vi "Interpolate 1D Array Main Page.vi"(8 "error in (no error)":errorcluster, 11 "Node Ptr":T5 format="%.0x") -> (0 "error out":errorcluster)   [LabVIEW 2011, in "Interpolate 1D Array Custom Device.lvlib"]
uses:
  Interpolate 1D Array Custom Device.lvlib
  <vilib>/NI Veristand/Custom Device API/Custom Device Item Ref.ctl
  Interpolate Options.ctl
  File Dependency Control.ctl
  <vilib>/NI Veristand/Custom Device API/Path Type.ctl
  Delimiter Control.ctl
  Spreadsheet Info.ctl
  <vilib>/NI Veristand/Custom Device API/Custom Device File Dependency.ctl
  <vilib>/NI Veristand/Custom Device API/Path Specification.ctl
  <vilib>/NI Veristand/Custom Device API/Custom Device Supported Target.ctl
  Global Property Names.vi
  <vilib>/NI Veristand/Custom Device API/Get Item Property (Variant).vi
  <vilib>/NI Veristand/Custom Device API/Set Item Property (Variant).vi
  <vilib>/NI Veristand/Custom Device API/Set Item Property (Path).vi
  <vilib>/NI Veristand/Custom Device API/Custom Device API.lvlib
panel:
  in  "Delimiter":T1
  in  "Dependency":T2={"Source"={"Local Path"=path "", "Type"=enum."Absolute"}, "RT Path"=path "", "Force Download File?"=TRUE}
  in  "Interpolate Options":T4={"method"=1, "ntimes"=1, "X is monotonic"=FALSE} {"method" items=["nearest", "linear", "spline", "cubic Hermite", "Lagrange"]}
  in  "Row Offset":dbl
  in  "Header":cluster{"Section Name":string}={"Section Name"="Custom Device Item Settings"}
  in  "Description":string
  in  "Name":string
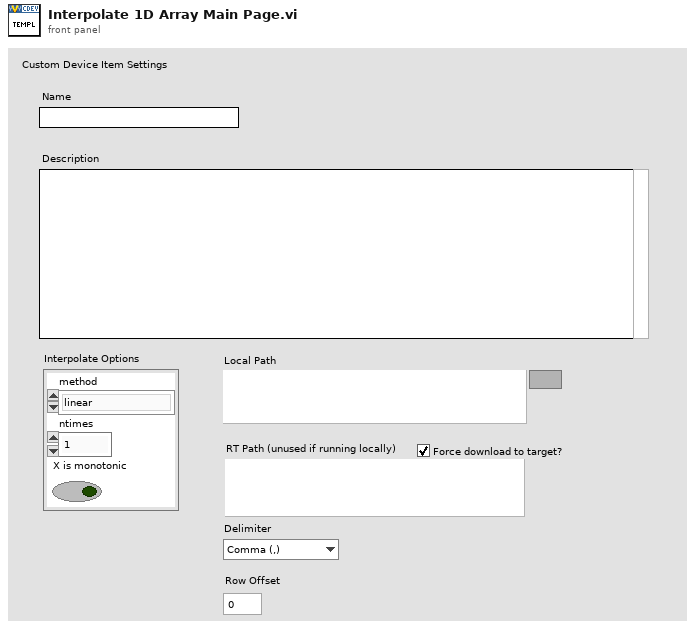
[diagram p1: front panel]
types:
  T1 = typedef "Interpolate 1D Array Custom Device.lvlib/Delimiter Control.ctl" = enum16{"Comma (,)", "Tab (\\t)"}
  T2 = typedef "Interpolate 1D Array Custom Device.lvlib/File Dependency Control.ctl" = cluster{"Source":cluster{"Local Path":path, "Type":T3}, "RT Path":path, "Force Download File?":bool}
  T3 = typedef "Custom Device API.lvlib/Path Type.ctl" = enum16{"Absolute", "To Base", "To Common Data Dir", "To Application Data Dir"}
  T4 = typedef "Interpolate 1D Array Custom Device.lvlib/Interpolate Options.ctl" = cluster{"method":i32, "ntimes":i32, "X is monotonic":bool}
  T5 = typedef "Custom Device API.lvlib/Custom Device Item Ref.ctl" = u64
  T6 = typedef "Interpolate 1D Array Custom Device.lvlib/Spreadsheet Info.ctl" = cluster{"Delimiter":string, "Row Offset":dbl}
  T7 = typedef "Custom Device API.lvlib/Custom Device File Dependency.ctl" = cluster{"Source":T8, "RT Destination":path, "ForceDownload?":bool, "SupportedTarget":T9, "Version":string}
  T8 = typedef "Custom Device API.lvlib/Path Specification.ctl" = cluster{"Path":path, "Type":T3}
  T9 = typedef "Custom Device API.lvlib/Custom Device Supported Target.ctl" = enum16{"All", "PharLap", "VxWorks", "Windows", "PharLap & Windows", "PharLap & VxWorks", "VxWorks & Windows"}
  T10 = typedef "Custom Device API.lvlib/Custom Device Item Info.ctl" = cluster{"Name":string, "Is Channel":bool, "GUID":string}
  T11 = typedef "Custom Device API.lvlib/Custom Device Commands.ctl" = enum16{"Default", "Item renamed", "Shutdown", "Dynamic button pressed"}
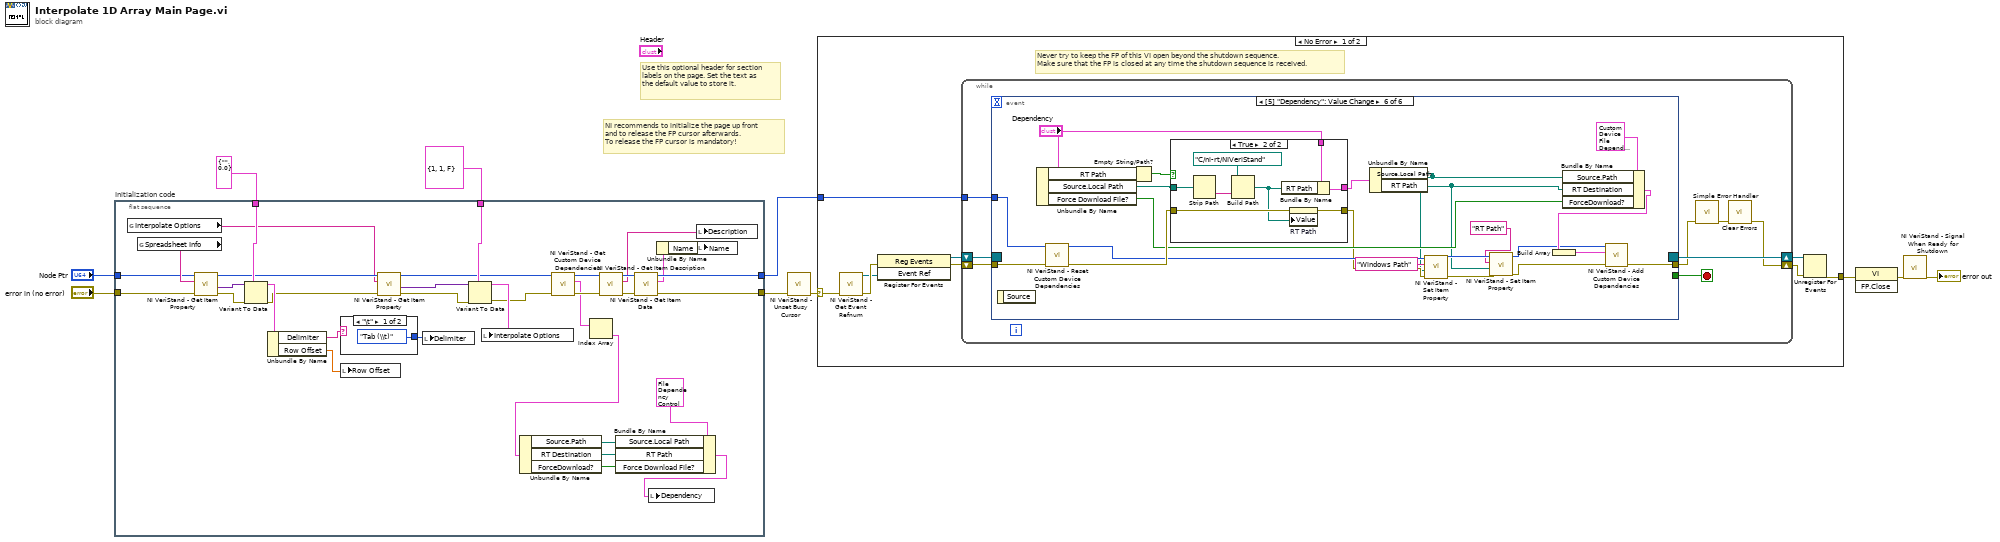
[diagram p0: block diagram]
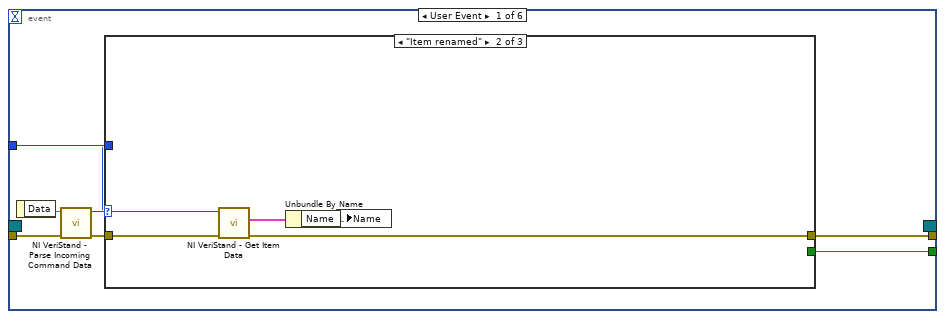
[diagram p2: hidden frame]
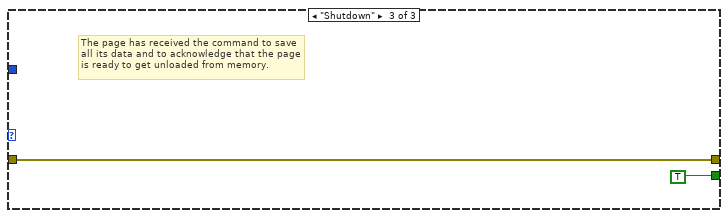
[diagram p4: hidden frame]
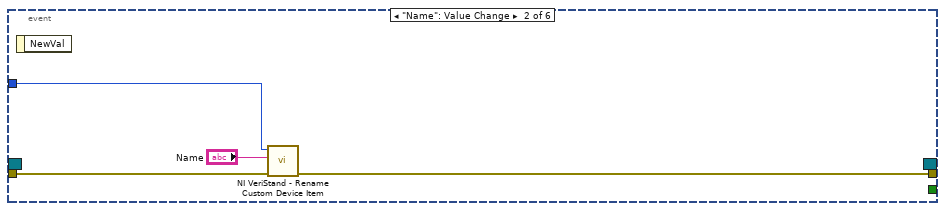
[diagram p5: hidden frame]
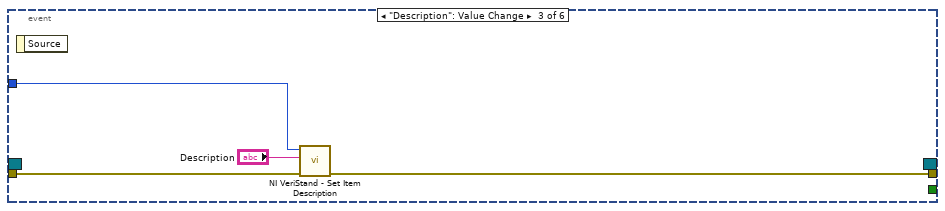
[diagram p6: hidden frame]
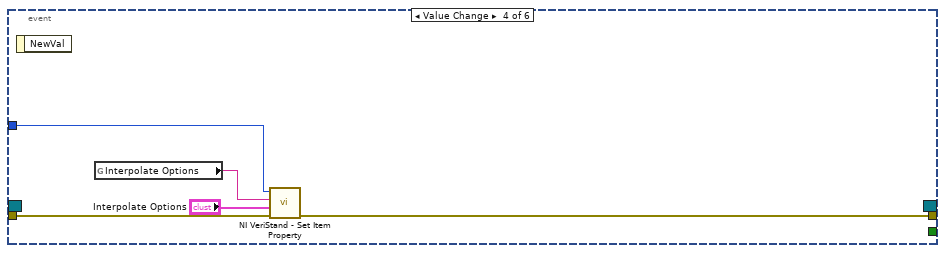
[diagram p7: hidden frame]
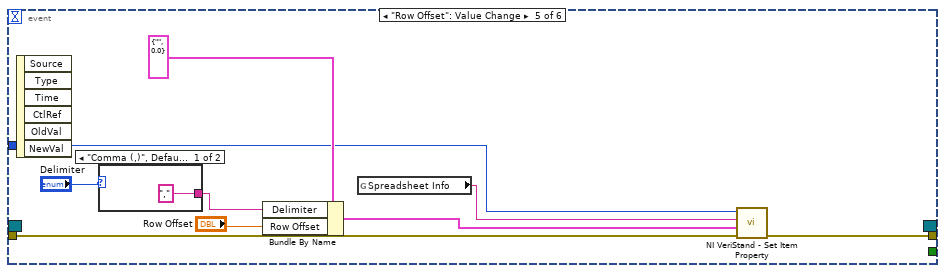
[diagram p8: hidden frame]
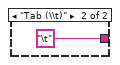
[diagram p9: hidden frame]
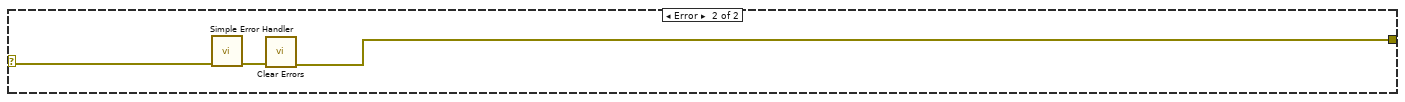
[diagram p11: hidden frame]
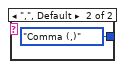
[diagram p12: hidden frame]
diagram:
  # "Use this optional header for section labels on the page. Set the text as the default value to store it."
  # "NI recommends to initialize the page up front\nand to release the FP cursor afterwards.\nTo release the FP cursor is mandatory!"
  n1 = flat-sequence "Initialization code" {
    tunnel: "error in (no error)" -> [w36]
    tunnel: "Node Ptr" -> [w37]
    tunnel: [w39] -> w8
    tunnel: [w45] -> w5
    tunnel: T6 {"Delimiter"="", "Row Offset"=0.0} ("Spreadsheet Info") -> [w33]
    tunnel: T4 {"method"=1, "ntimes"=1, "X is monotonic"=FALSE} ("Interpolate Options") -> [w26]
    frame #0 {
      n2 = global read "Global Property Names.vi" "Interpolate Options"() -> (w24:string)
      n3 = global read "Global Property Names.vi" "Spreadsheet Info"() -> (w38:string)
      n4 = call-poly <vilib>:"NI VeriStand - Get Item Property.vi"("error in (no error)"=w36, "Property Name"=w38, "Item Ref in"=w37) -> ("error out"=w34:errorcluster, "Value"=w35:variant, "Item Ref out"=w30:T5)  [unwired: 5 in, 1 out]
      n5 = Variant To Data(error in=w34, type=w33, Variant=w35) -> (data=w32:T6, error out=w29:errorcluster)
      n6 = Unbundle By Name(w32) -> ("Delimiter"=w18:string, "Row Offset"=w31:dbl)
      n7 = local write "Row Offset"(w31) -> ()
      n8 = case shown="\"\\t\"" w18 {
        tunnel: [Delimiter_Control."Tab (\\t)" ("Delimiter") Delimiter_Control."Comma (,)" ("Delimiter")] -> w17
        frame "\t" {
        }
        frame ",", Default {
        }
      }
      n9 = call-poly <vilib>:"NI VeriStand - Get Item Property.vi"("error in (no error)"=w29, "Property Name"=w24, "Item Ref in"=w30) -> ("error out"=w28:errorcluster, "Value"=w27:variant, "Item Ref out"=w22:T5)  [unwired: 5 in, 1 out]
      n10 = local write "Delimiter"(w17) -> ()
      n11 = Variant To Data(error in=w28, type=w26, Variant=w27) -> (data=w25:T4, error out=w23:errorcluster)
      n12 = local write "Interpolate Options"(w25) -> ()
      n13 = call <vilib>:"NI VeriStand - Get Custom Device Dependencies.vi"("error in (no error)"=w23, "Device Ref in"=w22) -> ("error out"=w20:errorcluster, "Dependencies"=w19:T7[], "Device Ref out"=w21:T5)  [unwired: 7 in]
      n14 = Index Array(array=w19) -> (element=w13:T7)  [unwired: 1 in]
      n15 = Unbundle By Name(w13) -> ("Source.Path"=w16:path, "RT Destination"=w14:path, "ForceDownload?"=w15:bool)
      n16 = call <vilib>:"NI VeriStand - Get Item Description.vi"("error in (no error)"=w20, "Item Ref in"=w21) -> ("error out"=w42:errorcluster, "Description"=w43:string, "Item Ref out"=w44:T5)  [unwired: 7 out]
      n17 = Bundle By Name(cluster=T2 {"Source"={"Local Path"=path "", "Type"=enum."Absolute"}, "RT Path"=path "", "Force Download File?"=TRUE} ("Dependency"), "Source.Local Path"=w16, "RT Path"=w14, "Force Download File?"=w15) -> (w12:T2)
      n18 = call <vilib>:"NI VeriStand - Get Item Data.vi"("error in (no error)"=w42, "Item Ref in"=w44) -> ("error out"=w39:errorcluster, "Item Info"=w41:T10, "Item Ref out"=w45:T5)  [unwired: 7 out]
      n19 = local write "Dependency"(w12) -> ()
      n20 = Unbundle By Name(w41) -> ("Name"=w40:string)
      n21 = local write "Description"(w43) -> ()
      n22 = local write "Name"(w40) -> ()
    }
  }
  n23 = call <vilib>:"NI VeriStand - Unset Busy Cursor.vi"("error in (no error)"=w8) -> ("error out"=w7:errorcluster)  [unwired: 10 out]
  n24 = case shown="No Error" w7 {
    selector: w7 -> [w48 w139]
    tunnel: [w53 w137] -> w10
    tunnel: w5 -> [w49 _]
    frame No Error {
      # "Never try to keep the FP of this VI open beyond the shutdown sequence.\nMake sure that the FP is closed at any time the shutdown sequence is received."
      n25 = call <vilib>:"NI VeriStand - Get Event Refnum.vi"("error in (no error)"=w48) -> ("error out"=w56:errorcluster, "Event Ref"=w52:refnum<user-event>)  [unwired: 9 out]
      n26 = register-events(error in=w56, w52) -> (reference out=w50:refnum<event-registration>, error out=w51:errorcluster)  [unwired: 1 in]
      n27 = while {
        tunnel: w49 -> [w60]
        shift-right: [w57] -> w54
        shift-left: w51 -> [w63]
        shift-right: [w64] -> w55
        shift-left: w50 -> [w62]
        stop <- w61 stop-if-true
        n28 = event shown="[5] \"Dependency\": Value Change" {
          selector: w62 -> [_ _ _ _ _ _]
          dyn-events: [_ _ _ _ _ _] -> w64
          timeout: _ -> [_ _ _ _ _ _]
          tunnel: w63 -> [w71 w83 w86 w91 w100 w123]
          tunnel: [w67 _ _ _ _ _] -> w61
          tunnel: [w66 w82 w85 w90 w99 w124] -> w59
          tunnel: w60 -> [w65 w81 w87 w92 w98 w126]
          event User Event {
            n29 = event-data() -> ("Data"=w70:string)  [unwired: 1 out]
            n30 = call <vilib>:"NI VeriStand - Parse Incoming Command Data.vi"("error in (no error)"=w71, "Incoming data"=w70) -> ("error out"=w69:errorcluster, "Action"=w68:T11)  [unwired: 8 out]
            n31 = case shown="\"Item renamed\"" w68 {
              tunnel: w69 -> [w72 w77 w78]
              tunnel: [_ _ TRUE] -> w67
              tunnel: [w72 w74 w78] -> w66
              tunnel: w65 -> [_ w76 _]
              frame "Default", Default {
              }
              frame "Item renamed" {
                n32 = call <vilib>:"NI VeriStand - Get Item Data.vi"("error in (no error)"=w77, "Item Ref in"=w76) -> ("error out"=w74:errorcluster, "Item Info"=w75:T10)  [unwired: 8 out]
                n33 = Unbundle By Name(w75) -> ("Name"=w73:string)
                n34 = local write "Name"(w73) -> ()
              }
              frame "Shutdown" {
                # "The page has received the command to save all its data and to acknowledge that the page is ready to get unloaded from memory."
              }
            }
          }
          event "Name": Value Change {
            n35 = event-data() -> ()  [unwired: 2 out]
            n36 = call <vilib>:"NI VeriStand - Rename Custom Device Item.vi"("error in (no error)"=w83, "New Name"="Name", "Item Ref in"=w81) -> ("error out"=w82:errorcluster)  [unwired: 8 out]
          }
          event "Description": Value Change {
            n37 = event-data() -> ()  [unwired: 2 out]
            n38 = call <vilib>:"NI VeriStand - Set Item Description.vi"("error in (no error)"=w86, "Description"="Description", "Item Ref in"=w87) -> ("error out"=w85:errorcluster)  [unwired: 8 out]
          }
          event Value Change {
            n39 = event-data() -> ()  [unwired: 2 out]
            n40 = global read "Global Property Names.vi" "Interpolate Options"() -> (w88:string)
            n41 = call-poly <vilib>:"NI VeriStand - Set Item Property.vi"("error in (no error)"=w91, "Value"="Interpolate Options", "Property Name"=w88, "Item Ref in"=w92) -> ("error out"=w90:errorcluster)  [unwired: 5 in, 2 out]
          }
          event "Row Offset": Value Change {
            n42 = event-data() -> ()  [unwired: 7 out]
            n43 = case shown="\"Comma (,)\", Default" "Delimiter" {
              tunnel: ["," ("Delimiter") "\t" ("Delimiter")] -> w93
              frame "Comma (,)", Default {
              }
              frame "Tab (\\t)" {
              }
            }
            n44 = Bundle By Name(cluster=T6 {"Delimiter"="", "Row Offset"=0.0} ("Spreadsheet Info"), "Delimiter"=w93, "Row Offset"="Row Offset") -> (w97:T6)
            n45 = global read "Global Property Names.vi" "Spreadsheet Info"() -> (w95:string)
            n46 = call-poly <vilib>:"NI VeriStand - Set Item Property.vi"("error in (no error)"=w100, "Value"=w97, "Property Name"=w95, "Item Ref in"=w98) -> ("error out"=w99:errorcluster)  [unwired: 5 in, 2 out]
          }
          event Value Change {
            n47 = event-data() -> ()  [unwired: 2 out]
            n48 = Unbundle By Name("Dependency") -> ("RT Path"=w122:path, "Source.Local Path"=w120:path, "Force Download File?"=w114:bool)
            n49 = call <vilib>:"NI VeriStand - Reset Custom Device Dependencies.vi"("error in (no error)"=w123, "Device Ref in"=w126) -> ("error out"=w118:errorcluster, "Device Ref out"=w113:T5)  [unwired: 8 in]
            n50 = Empty String/Path?(string/path=w122) -> (empty?=w121:bool)
            n51 = case shown="True" w121 {
              tunnel: "Dependency" -> [w128 w134]
              tunnel: [w128 w133] -> w115
              tunnel: w118 -> [w127 w131]
              tunnel: [w127 w130] -> w112
              tunnel: w120 -> [_ w132]
              frame False {
                # "Use the already specified path"
              }
              frame True {
                n52 = Strip Path(path=w132) -> (name=w135:string)  [unwired: 1 out]
                n53 = Build Path(base path=path "C:/ni-rt/NIVeriStand", name or relative path=w135) -> (appended path=w129:path)
                n54 = Bundle By Name(cluster=w134, "RT Path"=w129) -> (w133:T2)
                n55 = property on="RT Path" class="Path"(error in=w131, "Value"=w129) -> (error out=w130:errorcluster)  [unwired: 1 in, 1 out]
              }
            }
            n56 = Unbundle By Name(w115) -> ("Source.Local Path"=w106:path, "RT Path"=w104:path)
            n57 = call-poly <vilib>:"NI VeriStand - Set Item Property.vi"("error in (no error)"=w112, "Value"=w106, "Property Name"="Windows Path", "Item Ref in"=w113) -> ("error out"=w111:errorcluster, "Item Ref out"=w108:T5)  [unwired: 5 in, 1 out]
            n58 = call-poly <vilib>:"NI VeriStand - Set Item Property.vi"("error in (no error)"=w111, "Value"=w104, "Property Name"="RT Path", "Item Ref in"=w108) -> ("error out"=w110:errorcluster, "Item Ref out"=w109:T5)  [unwired: 5 in, 1 out]
            n59 = Bundle By Name(cluster=T7 {"Source"={"Path"=path "", "Type"=enum."Absolute"}, "RT Destination"=path "", "ForceDownload?"=FALSE, "SupportedTarget"=enum."PharLap", "Version"=""} ("Dependency"), "Source.Path"=w106, "RT Destination"=w104, "ForceDownload?"=w114) -> (w116:T7)
            n60 = Build Array(w116) -> (w125:T7[])
            n61 = call <vilib>:"NI VeriStand - Add Custom Device Dependencies.vi"("error in (no error)"=w110, "Dependencies"=w125, "Device Ref in"=w109) -> ("error out"=w124:errorcluster)  [unwired: 8 out]
          }
        }
        n62 = call <vilib>:"Simple Error Handler.vi"("error in (no error)"=w59) -> ("error out"=w58:errorcluster)  [unwired: 1 in, 7 out]
        n63 = call <vilib>:"Clear Errors.vi"("error in (no error)"=w58) -> ("error out"=w57:errorcluster)  [unwired: 6 out]
      }
      n64 = Unregister For Events(event registration refnum=w55, error in=w54) -> (error out=w53:errorcluster)
    }
    frame Error {
      n65 = call <vilib>:"Simple Error Handler.vi"("error in (no error)"=w139) -> ("error out"=w138:errorcluster)  [unwired: 1 in, 7 out]
      n66 = call <vilib>:"Clear Errors.vi"("error in (no error)"=w138) -> ("error out"=w137:errorcluster)  [unwired: 6 out]
    }
  }
  n67 = invoke class="VI" method="FP.Close"(error in=w10) -> (error out=w2:errorcluster)  [unwired: 2 in, 2 out]
  n68 = call <vilib>:"NI VeriStand - Signal When Ready for Shutdown.vi"("error in (no error)"=w2) -> ("error out"=→"error out":errorcluster)  [unwired: 10 out]
